vi "Bitfield_Replace.vi"(5 "stop":u8, 7 "start":u8, 10 "value new (In)":u32=7 format="%032b", 11 "value old (In)":u32=12690 format="%032b") -> (3 "value (Out)":u32 format="%032b")   [LabVIEW 2014]
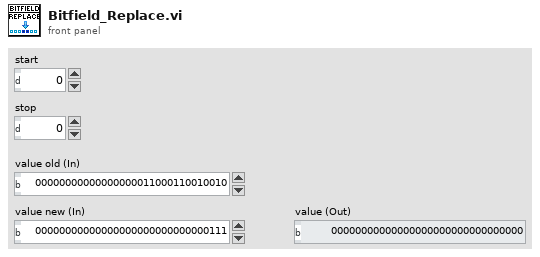
[diagram p1: front panel]
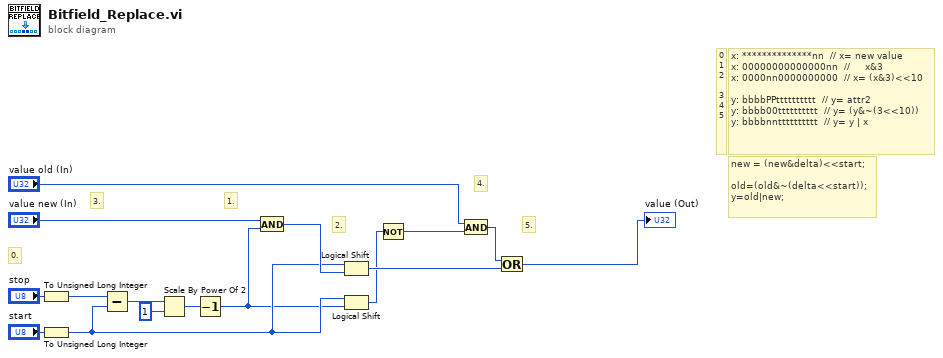
[diagram p0: block diagram]
diagram:
  # "3."
  # "5."
  # "4."
  # "new = (new&delta)<<start;\n\nold=(old&~(delta<<start));\ny=old|new;"
  # "2."
  # "1."
  # "0."
  # "0\n1\n2\n\n3\n4\n5"
  # "x: **************nn  // x= new value\nx: 00000000000000nn  //     x&3\nx: 0000nn0000000000  // x= (x&3)<<10\n\ny: bbbbPPtttttttttt  // y= attr2\ny: bbbb00tttttttttt  // y= (y&~(3<<10))\ny: bbbbnntttttttttt  // y= y | x"
  n1 = To Unsigned Long Integer(number="stop") -> (unsigned 32bit integer=w10:u32)
  n2 = To Unsigned Long Integer(number="start") -> (unsigned 32bit integer=w6:u32)
  n3 = Subtract(x=w10, y=w6) -> (x-y=w7:u32)
  n4 = Scale By Power Of 2(n=w7, x=u32 1) -> (x*2^n=w8:u32)
  n5 = Decrement(x=w8) -> (x-1=w4:u32)
  n6 = And(x="value new (In)", y=w4) -> (x .and. y?=w13:u32)
  n7 = Logical Shift(y=w6, x=w13) -> (x << y=w12:u32)
  n8 = Logical Shift(y=w6, x=w4) -> (x << y=w3:u32)
  n9 = Not(x=w3) -> (.not. x?=w5:u32)
  n10 = And(x="value old (In)", y=w5) -> (x .and. y?=w9:u32)
  n11 = Or(x=w9, y=w12) -> (x .or. y?=→"value (Out)":u32)
